vi "Log Info.vi"(2 "EnableLogging?":bool, 5 "Message":string) -> ()   [LabVIEW 2020, in "TaskfileRunner Tool.lvlib"]
doc: "Add a info message to the log"
uses:
  TaskfileRunner Tool.lvlib
  3b7a71ad-25d6-447f-a954-168ecec1f7c2.vi
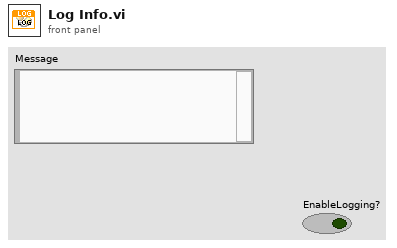
[diagram p1: front panel]
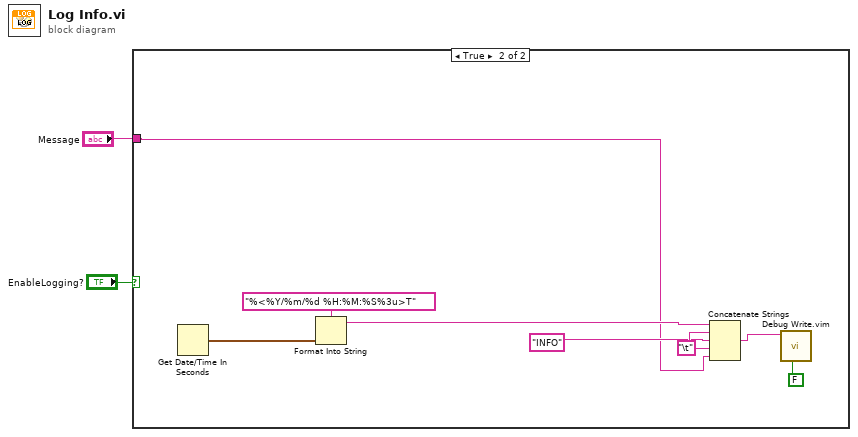
[diagram p0: block diagram]
diagram:
  n1 = case shown="True" "EnableLogging?" {
    tunnel: "Message" -> [_ w3]
    frame False {
    }
    frame True {
      w6 = "\t"
      n2 = Get Date/Time In Seconds() -> (seconds since 1Jan1904=w10:timestamp)
      n3 = Format Into String(format string="%<%Y/%m/%d %H:%M:%S%3u>T", w10) -> (resulting string=w8:string)  [unwired: 2 in, 1 out]
      n4 = Concatenate Strings(w8, w6, "INFO", w6, w3) -> (w5:string)
      n5 = call "Debug Write.vim"("include timestamp? (F)"=FALSE, "value"=w5) -> ()  [unwired: 9 in, 1 out]
    }
  }
